vi "myPID_waveform.vi"() -> ()   [LabVIEW 2018]
panel:
  in  "Stop Button":bool
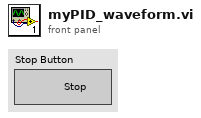
[diagram p1: front panel]
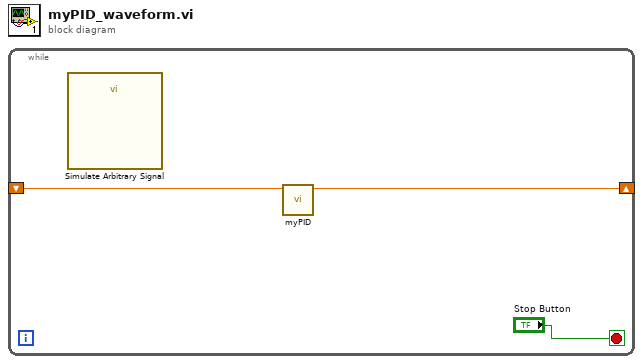
[diagram p0: block diagram]
diagram:
  n1 = while {
    shift-right: [w2] -> _
    shift-left: _ -> [w1]
    stop <- "Stop Button" stop-if-true
    n2 = call "Simulate Arbitrary Signal"() -> ()  [unwired: 9 in, 3 out]
    n3 = call "myPID.vi"("Numeric"=w1) -> ("Numeric 2"=w2:dbl)  [unwired: 10 in]
  }
